vi "Run.vi"(8 "error in (no error)":errorcluster, 11 "PmuDelayClass in":refnum<class "FreqAnalysis.lvclass">) -> (0 "error out":errorcluster, 2 "TimeOut":bool, 3 "PmuDelayClass out":refnum<class "FreqAnalysis.lvclass">)   [LabVIEW 2018, in "AnalysisPlugins.lvlib" / "FreqAnalysis.lvclass"]
uses:
  FreqAnalysis.lvclass
  C:/projects/ICDAS/NistPluggableModules/Analysis/AnalysisPlugins/AnalysisPluginBaseClass/AnalysisPluginsBase.lvclass
  C:/projects/ICDAS/NistPluggableModules/Analysis/AnalysisPlugins/FitterBaseClass/FitterBase.lvclass
  AnalysisPluginBaseClass/AnalysisPluginsBase.lvclass/AnalysisPluginsBase.ctl
  AnalysisPluginBaseClass/Accessors/Read Duration.vi
  AnalysisPluginBaseClass/Accessors/Read AnalysisTime.vi
  AnalysisPluginBaseClass/Accessors/Read Window.vi
  FitterBaseClass/FitterBase.lvclass
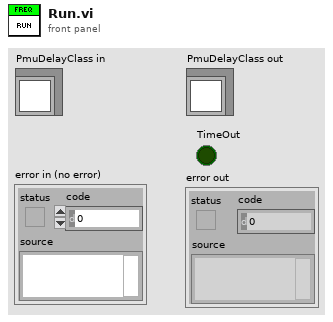
[diagram p1: front panel]
types:
  T1 = typedef "AnalysisPlugins.lvlib/AnalysisPluginsBase.lvclass/clWindowData.ctl" = cluster{"Timestamp":ext, "Samples":dbl[][], "Window Valid":bool, "T0":ext}
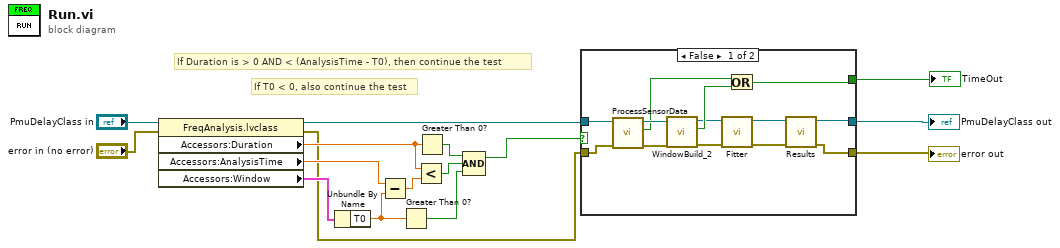
[diagram p0: block diagram]
diagram:
  # "If T0 < 0, also continue the test"
  # "If Duration is > 0 AND < (AnalysisTime - T0), then continue the test"
  n1 = property class="FreqAnalysis.lvclass"(reference="PmuDelayClass in", error in="error in (no error)") -> (reference out=w2:refnum<class "FreqAnalysis.lvclass">, error out=w1:errorcluster, "Accessors:Duration"=w11:dbl, "Accessors:AnalysisTime"=w9:dbl, "Accessors:Window"=w7:T1)
  n2 = Unbundle By Name(w7) -> ("T0"=w8:ext)
  n3 = Subtract(x=w9, y=w8) -> (x-y=w10:ext)
  n4 = Greater Than 0?(x=w8) -> (x > 0?=w4:bool)
  n5 = Less?(x=w11, y=w10) -> (x < y?=w5:bool)
  n6 = Greater Than 0?(x=w11) -> (x > 0?=w6:bool)
  n7 = Compound Arithmetic op=AND(w6, w5, w4) -> (w3:bool)
  n8 = case shown="False" w3 {
    selector: w3 -> [_ w31]
    tunnel: w1 -> [w29 w32]
    tunnel: [w19 w32] -> w16
    tunnel: [w20 w31] -> w15
    tunnel: [w17 w30] -> w14
    tunnel: w2 -> [w18 w30]
    frame False {
      n9 = call-dynamic "ProcessSensorData.vi"("error in (no error)"=w29, "PmuAnalysis"=w18) -> ("error out"=w27:errorcluster, "TimedOut"=w26:bool, "PMUAnalysis"=w28:refnum<class "FreqAnalysis.lvclass">)  [unwired: 7 in]
      n10 = call "WindowBuild_2.vi"("Error In"=w27, "Fitter in"=w28) -> ("Error Out"=w23:errorcluster, "Timeout"=w25:bool, "Fitter out"=w24:refnum<class "FreqAnalysis.lvclass">)  [unwired: 7 in]
      n11 = call-dynamic "Fitter.vi"("error in (no error)"=w23, "PmuAnalysis in"=w24) -> ("error out"=w22:errorcluster, "PmuAnalysis out"=w21:refnum<class "FreqAnalysis.lvclass">)  [unwired: 8 in]
      n12 = Or(x=w26, y=w25) -> (x .or. y?=w20:bool)
      n13 = call-dynamic "Results.vi"("error in (no error)"=w22, "PmuDelayClass in"=w21) -> ("error out"=w19:errorcluster, "PmuDelayClass out"=w17:refnum<class "FreqAnalysis.lvclass">)  [unwired: 8 in]
    }
    frame True {
    }
  }
  "error out" <- w16
  "PmuDelayClass out" <- w14
  "TimeOut" <- w15
